vi "set initial camera config.vi"(8 "error in (no error)":errorcluster, 11 "ECHARPE_Channel in":refnum<class "ECHARPE_Channel.lvclass">) -> (0 "error out":errorcluster, 3 "ECHARPE_Channel out":refnum<class "ECHARPE_Channel.lvclass">)   [LabVIEW 2018, in "ECHARPE_Channel.lvclass"]
uses:
  ECHARPE_Channel.lvclass
  Sim_CCD/Sim_CCD.lvclass
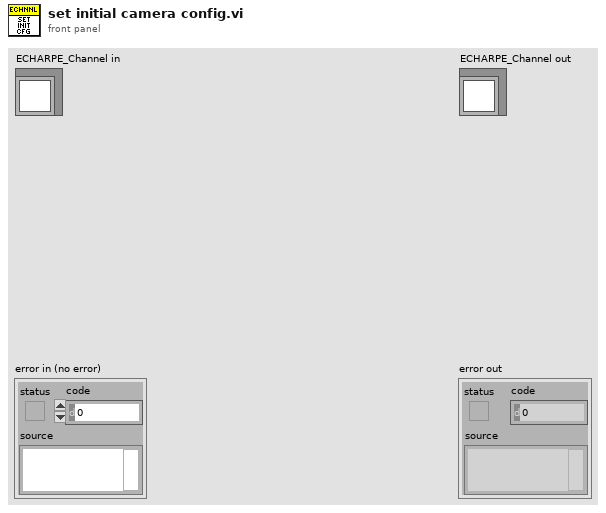
[diagram p1: front panel]
types:
  T1 = cluster{"PREAMP":u16, "READOUT_RATE":u16, "VERTICAL_SHIFT_SPEED":u16, "READ_MODE":u16, "VERTICAL_CLOCK_VOLTAGE":u16, "ACQUISITION_MODE":u16, "AD_CHANNEL":u16, "SHUTTER_TTL":u16, "SHUTTER_OPENING_TIME":u16, "SHUTTER_CLOSING_TIME":u16, "SHUTTER_MODE":u16, "TRIGGER_MODE":u16, "VBIN":u16, "INITIAL_LINE":u16, "INITIAL_COLUMN":u16, "FINAL_LINE":u16, "FINAL_COLUMN":u16, "HBIN":u16}
  T2 = cluster{"State Machine.lvclass":refnum<class "State Machine.lvclass">, "RxTx.lvclass":refnum<class "RxTx.lvclass">, "Save_Header_RxTx.lvclass":refnum<class "RxTx.lvclass">, "Status SM.lvclass":refnum<class "State Machine.lvclass">, "Status RxTx.lvclass":refnum<class "RxTx.lvclass">, "servers array":refnum<class "Server.lvclass">[], "Events log file.lvclass":refnum<class "Log File.lvclass">, "Errors log file.lvclass":refnum<class "Log File.lvclass">, "Keywords log file.lvclass":refnum<class "Log File.lvclass">, "Sim_CCD.lvclass":refnum<class "Sim_CCD.lvclass">}
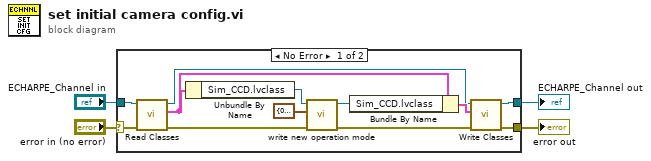
[diagram p0: block diagram]
diagram:
  n1 = case shown="No Error" "error in (no error)" {
    selector: "error in (no error)" -> [w7 w17]
    tunnel: "ECHARPE_Channel in" -> [w8 w18]
    tunnel: [w6 w18] -> w2
    tunnel: [w5 w17] -> w1
    frame No Error {
      n2 = call-dynamic "Read Classes.vi"("error in (no error)"=w7, "Channel in"=w8) -> ("error out"=w12:errorcluster, "Classes"=w16:T2, "Channel out"=w9:refnum<class "ECHARPE_Channel.lvclass">)  [unwired: 7 in]
      n3 = Unbundle By Name(w16) -> ("Sim_CCD.lvclass"=w14:refnum<class "Sim_CCD.lvclass">)
      n4 = call "write new operation mode.vi"("error in (no error)"=w12, "new operation mode"=T1 {"PREAMP"=0, "READOUT_RATE"=0, "VERTICAL_SHIFT_SPEED"=0, "READ_MODE"=4, "VERTICAL_CLOCK_VOLTAGE"=0, "ACQUISITION_MODE"=3, "AD_CHANNEL"=0, "SHUTTER_TTL"=0, "SHUTTER_OPENING_TIME"=50, "SHUTTER_CLOSING_TIME"=50, "SHUTTER_MODE"=2, "TRIGGER_MODE"=0, "VBIN"=1, "INITIAL_LINE"=1, "INITIAL_COLUMN"=1, "FINAL_LINE"=1024, "FINAL_COLUMN"=1024, "HBIN"=1} ("prev operation mode 2"), "CCDCamera in"=w14) -> ("error out"=w11:errorcluster, "CCDCamera out"=w13:refnum<class "Sim_CCD.lvclass">)  [unwired: 7 in]
      n5 = Bundle By Name(cluster=w16, "Sim_CCD.lvclass"=w13) -> (w15:T2)
      n6 = call-dynamic "Write Classes.vi"("error in (no error)"=w11, "Classes"=w15, "Channel in"=w9) -> ("error out"=w5:errorcluster, "Channel out"=w6:refnum<class "ECHARPE_Channel.lvclass">)  [unwired: 7 in]
    }
    frame Error {
    }
  }
  "error out" <- w1
  "ECHARPE_Channel out" <- w2
